vi "Get Ctrl Refnum.vi"(8 "error in (no error)":errorcluster, 11 "Field Configuration in":refnum<class "Field Configuration.lvclass">) -> (0 "error out":errorcluster, 2 "Ctl Refnum":refnum<vi>, 3 "Field Configuration out":refnum<class "Field Configuration.lvclass">)   [LabVIEW 2020, in "Field Interfaces.lvlib" / "Field Configuration.lvclass"]
uses:
  Field Configuration.lvclass
  Field Configuration.lvclass/Field Configuration.ctl
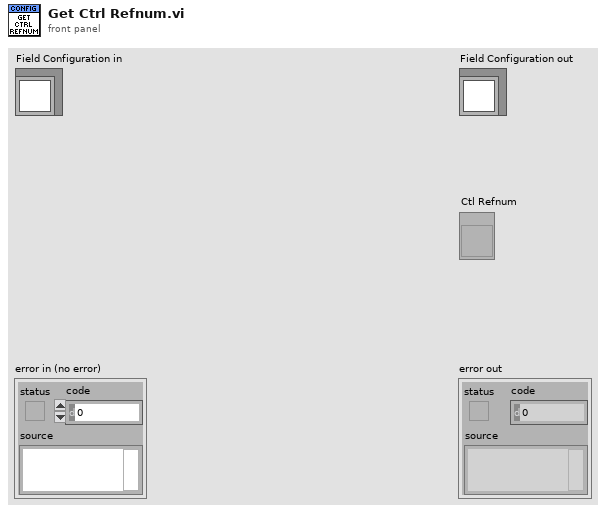
[diagram p1: front panel]
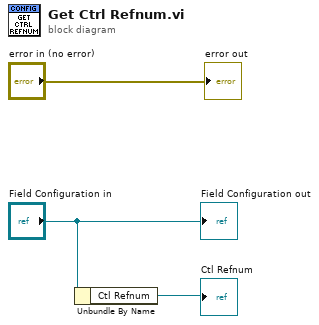
[diagram p0: block diagram]
diagram:
  n1 = Unbundle By Name("Field Configuration in") -> ("Ctl Refnum"=→"Ctl Refnum":refnum<vi>)
  "error out" <- "error in (no error)"
  "Field Configuration out" <- "Field Configuration in"
